vi "Lab Suma total de los valores de un arreglo-2.vi"() -> ()   [LabVIEW 2018]
panel:
  in  "Slide":dbl(slide) scale=0.0..10.0
  out "Numeric 2":dbl
  in  "stop":bool
  out "Numeric":dbl
  out "Array":dbl[](array[numeric])
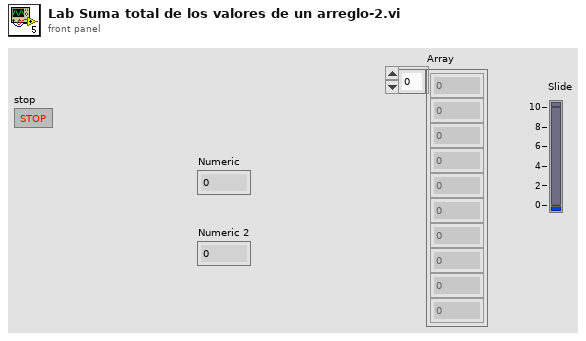
[diagram p1: front panel]
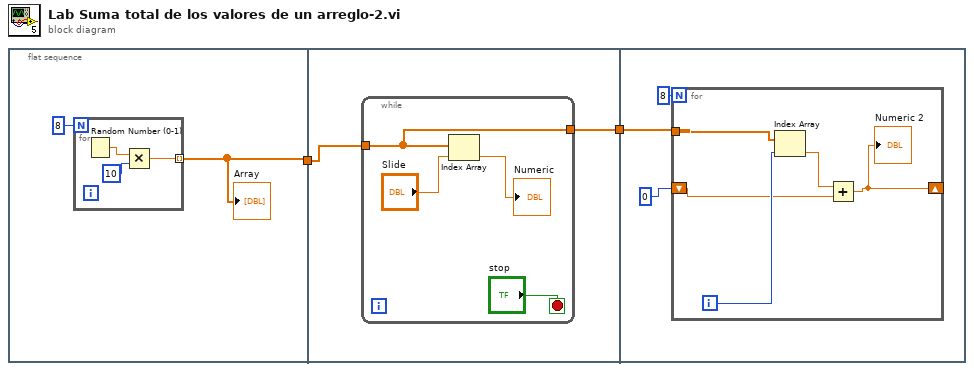
[diagram p0: block diagram]
diagram:
  n1 = flat-sequence {
    tunnel: [w3] -> w2
    tunnel: w2 -> [w9]
    tunnel: [w8] -> w1
    tunnel: w1 -> [w15]
    frame #0 {
      n2 = for {
        N: 8 -> [_]
        tunnel: [w5] -> w3 mode=indexing
        n3 = Random Number (0-1)() -> (number: 0 to 1=w7:dbl)
        n4 = Multiply(x=w7, y=10) -> (x*y=w5:dbl)
      }
      "Array" <- w3
    }
    frame #1 {
      n5 = while {
        tunnel: w9 -> [w11]
        tunnel: [w11] -> w8
        stop <- "stop" stop-if-true
        n6 = Index Array(array=w11, index="Slide") -> (element=→"Numeric":dbl)
      }
    }
    frame #2 {
      n7 = for {
        N: 8 -> [_]
        tunnel: w15 -> [w21]
        shift-right: [w17] -> _
        shift-left: 0 -> [w18]
        i -> [w20]
        n8 = Index Array(array=w21, index=w20) -> (element=w19:dbl)
        n9 = Add(x=w19, y=w18) -> (x+y=w17:dbl)
        "Numeric 2" <- w17
      }
    }
  }
